vi "제목없음 1.vi"() -> ()   [LabVIEW 2014]
uses:
  <vilib>/myRIO/Instrument Drivers/Onboard IO/AI/vis/Read.vi
  <vilib>/myRIO/Instrument Drivers/Onboard IO/AI/vis/Smart Open.vi
  <vilib>/Utility/error.llb/Error Cluster From Error Code.vi
  <vilib>/myRIO/Common/Instrument Driver Framework/myRIO v1.0/AI/vis/myRIO v1.0 Read AI.vi
panel:
  out "abs(x) 2":dbl
  out "abs(x)":dbl
  in  "Servo Position (0 - 255) 2":u8(slide)=128 step=1 scale=0.0..255.0
  in  "Servo Position (0 - 255)":u8(slide)=233 step=1 scale=0.0..255.0
  in  "숫자형 8":dbl=10.0
  in  "숫자형 7":dbl=10.0
  in  "숫자형 6":dbl=-10.0
  in  "숫자형 5":dbl=10.0
  in  "불리언 4":bool
  out "컬러센서2번 (B/AI2 (Pin 7))":dbl=2.614745826
  out "컬러센서1번 (B/AI1 (Pin 5))":dbl=2.67333957
  in  "숫자형 4":dbl
  out "컬러센서0번 (B/AI0 (Pin 3))":dbl=2.4340817820000002
  out "웨이브폼 차트":dbl(graph)=2.4340817820000002
  in  "불리언 2":bool=TRUE
  in  "숫자형 3":dbl=128.0
  in  "숫자형 2":dbl=122.0
  in  "숫자형":dbl=120.0
  in  "불리언 3":bool=TRUE
  in  "불리언":bool=TRUE
  in  "Controller Daisy Chain Position (1 - 4)":u8=1
  in  "정지":bool
  # "오른"
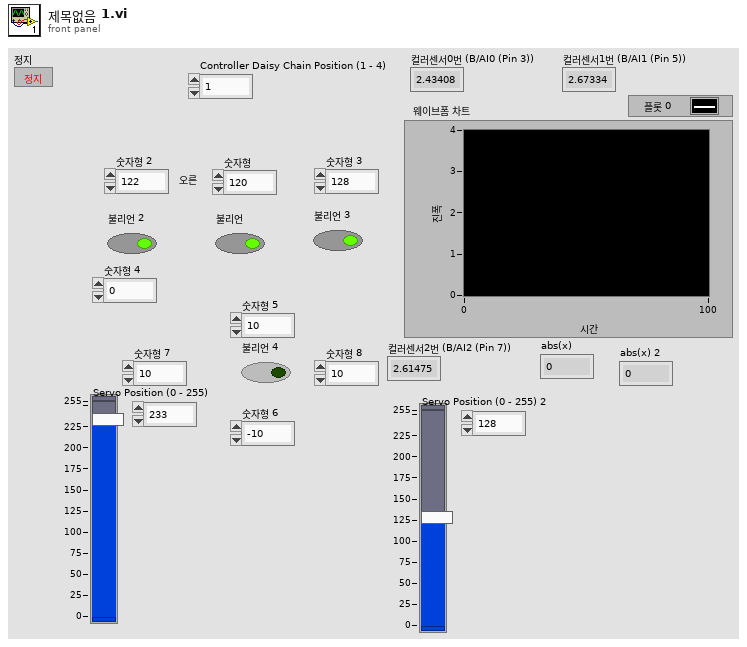
[diagram p1: front panel]
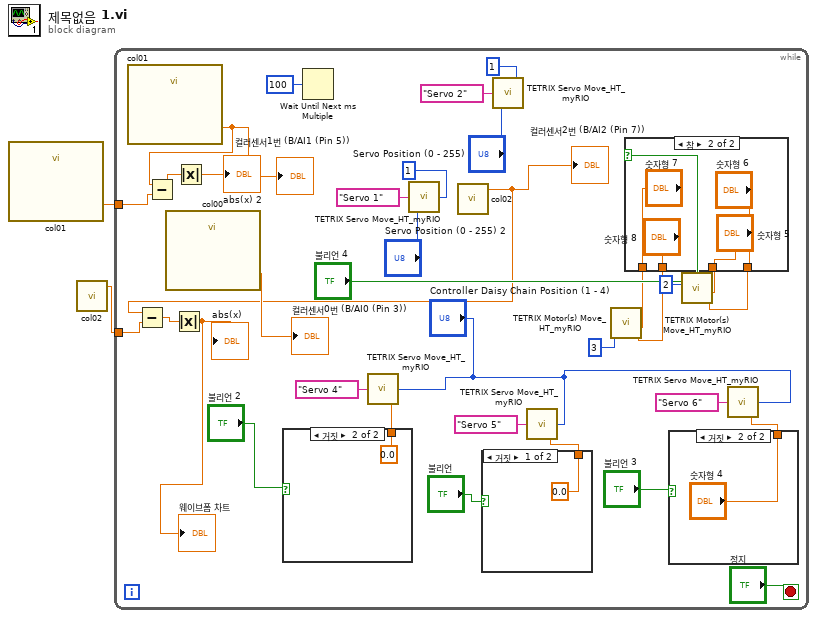
[diagram p0: block diagram]
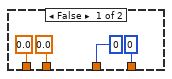
[diagram p2: hidden frame]
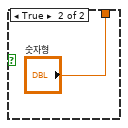
[diagram p3: hidden frame]
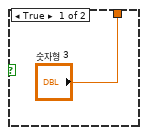
[diagram p4: hidden frame]
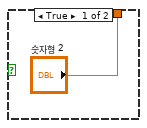
[diagram p5: hidden frame]
diagram:
  n1 = call "col01.vi"() -> ("Col01 (B/AI1 (Pin 5))"=w1:dbl)  [unwired: 26 in, 1 out]
  n2 = call "col02.vi"() -> ("Col02 (B/AI2 (Pin 7))"=w2:dbl)  [unwired: 26 in, 1 out]
  n3 = while {
    tunnel: w2 -> [w9]
    tunnel: w1 -> [w4]
    stop <- "정지" stop-if-true
    n4 = call "col01.vi"() -> ("Col01 (B/AI1 (Pin 5))"=w5:dbl)  [unwired: 26 in, 1 out]
    "컬러센서1번 (B/AI1 (Pin 5))" <- w5
    n5 = Subtract(x=w5, y=w4) -> (x-y=w6:dbl)
    n6 = call "col00.vi"() -> ("Col00 (B/AI0 (Pin 3))"=→"컬러센서0번 (B/AI0 (Pin 3))":dbl)  [unwired: 26 in, 1 out]
    n7 = Absolute Value(x=w6) -> (abs(x)=→"abs(x) 2":dbl)
    n8 = case shown="거짓" "불리언 2" {
      tunnel: ["숫자형 2" 0.0 ("슬라이드")] -> w32
      frame True {
      }
      frame False {
      }
    }
    n9 = Wait Until Next ms Multiple(millisecond multiple=u32 100 ("ms 배수")) -> ()  [unwired: 1 out]
    n10 = call <vilib>:"TETRIX Servo Move_HT_myRIO.vi"("Servo Position (0 - 255)"=w32, "Controller Daisy Chain Position (1 - 4)"="Controller Daisy Chain Position (1 - 4)", "Select Servo"="Servo 4") -> ()  [unwired: 2 in, 1 out]
    n11 = call <vilib>:"TETRIX Servo Move_HT_myRIO.vi"("Servo Position (0 - 255)"="Servo Position (0 - 255) 2", "Controller Daisy Chain Position (1 - 4)"=u8 1, "Select Servo"="Servo 1") -> ()  [unwired: 2 in, 1 out]
    n12 = call "col02.vi"() -> ("Col02 (B/AI2 (Pin 7))"=w10:dbl)  [unwired: 26 in, 1 out]
    "컬러센서2번 (B/AI2 (Pin 7))" <- w10
    n13 = Subtract(x=w10, y=w9) -> (x-y=w8:dbl)
    n14 = Absolute Value(x=w8) -> (abs(x)=→"웨이브폼 차트" →"abs(x)":dbl)
    n15 = case shown="거짓" "불리언" {
      tunnel: [0.0 ("슬라이드") "숫자형"] -> w28
      frame False {
      }
      frame True {
      }
    }
    n16 = call <vilib>:"TETRIX Servo Move_HT_myRIO.vi"("Servo Position (0 - 255)"="Servo Position (0 - 255)", "Controller Daisy Chain Position (1 - 4)"=u8 1, "Select Servo"="Servo 2") -> ()  [unwired: 2 in, 1 out]
    n17 = call <vilib>:"TETRIX Servo Move_HT_myRIO.vi"("Servo Position (0 - 255)"=w28, "Controller Daisy Chain Position (1 - 4)"="Controller Daisy Chain Position (1 - 4)", "Select Servo"="Servo 5") -> ()  [unwired: 2 in, 1 out]
    n18 = case shown="참" "불리언 4" {
      tunnel: [i8 0 ("Motor 1 Power (-100 to 100)\n0 = Stop/Brake\n-128 = Stop/Coast") "숫자형 5"] -> w22
      tunnel: [i8 0 ("Motor 1 Power (-100 to 100)\n0 = Stop/Brake\n-128 = Stop/Coast") "숫자형 6"] -> w21
      tunnel: [0.0 ("숫자형 8") "숫자형 8"] -> w18
      tunnel: [0.0 ("숫자형 7") "숫자형 7"] -> w17
      frame False {
      }
      frame True {
      }
    }
    n19 = call <vilib>:"TETRIX Motor(s) Move_HT_myRIO.vi"("Motor 2 Power (-100 to 100)\n0 = Stop/Brake\n-128 = Stop/Coast"=w18, "Motor 1 Power (-100 to 100)\n0 = Stop/Brake\n-128 = Stop/Coast"=w17, "Controller Daisy Chain Position: 1 - 4"=u8 3) -> ()  [unwired: 6 in, 1 out]
    n20 = case shown="거짓" "불리언 3" {
      tunnel: ["숫자형 3" "숫자형 4"] -> w30
      frame True {
      }
      frame False {
      }
    }
    n21 = call <vilib>:"TETRIX Motor(s) Move_HT_myRIO.vi"("Motor 2 Power (-100 to 100)\n0 = Stop/Brake\n-128 = Stop/Coast"=w21, "Motor 1 Power (-100 to 100)\n0 = Stop/Brake\n-128 = Stop/Coast"=w22, "Controller Daisy Chain Position: 1 - 4"=u8 2) -> ()  [unwired: 6 in, 1 out]
    n22 = call <vilib>:"TETRIX Servo Move_HT_myRIO.vi"("Servo Position (0 - 255)"=w30, "Controller Daisy Chain Position (1 - 4)"="Controller Daisy Chain Position (1 - 4)", "Select Servo"="Servo 6") -> ()  [unwired: 2 in, 1 out]
  }
